vi "Save_ADAM_Table_Locally.vi"   [LabVIEW 2013]
uses:
  ADAM Controls/Update_scan_value.ctl
  Anemometry/Anemometry Sub Vis/Controls/Global_mode.ctl
  Anemometry/Anemometry Sub Vis/Globals/Trav_pos_global.vi
types:
  T1 = typedef "Global_mode.ctl" = enum16{"Read Global", "Load Global From File", "Write Global to File"}
  T2 = typedef "Update_scan_value.ctl" = cluster{"Channel Name":string, "New Value":dbl}
  T3 = typedef "Ch_description_ADAM.ctl" = cluster{"Ch Name":string, "Type":T4, "Function":T5, "Ch State":T6, "Calibration type":T7, "A":dbl, "B":dbl, "C":dbl, "D":dbl, "Comments":string, "Address":T8, "String":string, "Duty":u16}
  T4 = typedef "Module_type_ADAM.ctl" = string
  T5 = typedef "Function_ADAM.ctl" = enum16{"Analogue Input", "Digital Input", "Event counter", "Event rate", "Analogue Output", "Digital Output", "Relay Output"}
  T6 = typedef "Channel_State.ctl" = enum16{"On", "Off", "Always On", "Always Off"}
  T7 = typedef "Calib_type_ADAM.ctl" = enum16{"Raw", "Bx + A", "Cx^2 + Bx + A", "Dx^3 + Cx^2 + Bx + A", "In Band", "Hi-Tec Q", "Hi-Tec M_dot", "Text"}
  T8 = typedef "Address.ctl" = cluster{"Main":i32, "Ch.":i32, "Sub":i32, "Port Name":string}
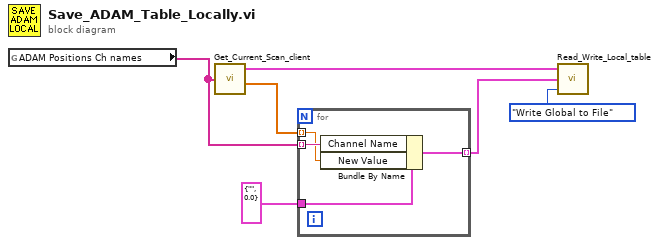
[diagram p0: block diagram]
diagram:
  n1 = global read "Trav_pos_global.vi" "ADAM Positions Ch names"() -> (w1:string[])
  n2 = call "Get_Current_Scan_client.vi"("ADAM Ch Names"=w1) -> ("Ch Description Array"=w6:T3[], "Numerical Values"=w4:dbl[])  [unwired: 1 in, 1 out]
  n3 = for {
    tunnel: T2 {"Channel Name"="", "New Value"=0.0} ("Update Scan Value Cluster") -> [w10]
    tunnel: w1 -> [w9] mode=indexing
    tunnel: w4 -> [w8] mode=indexing
    tunnel: [w7] -> w2 mode=indexing
    n4 = Bundle By Name(cluster=w10, "Channel Name"=w9, "New Value"=w8) -> (w7:T2)
  }
  n5 = call "Read_Write_Local_table.vi"("Mode"=Global_mode."Write Global to File", "Ch Values in"=w2, "Channels Descriptions In"=w6) -> ()  [unwired: 3 out]
